vi "WPI_ADI_IMU_RefNum Registry Get.vi"(8 "error in (no error)":errorcluster, 11 "refnum name":string="ADIIMURefNum") -> (0 "error out":errorcluster, 3 "ADI IMU Interrupt DevRef":T1={"SimpleGyroDevRef"={"DevStatus"={"status"=FALSE, "code"=0, "source"=""}, "Handle"=0, "SPI Bus"=enum."SPI On-Board, CS0", "Device Found"=FALSE, "Sample Rate"=0.0, "Device Ready"=FALSE, "Yaw Axis"=enum."Z", "AHRS Algorithm"=enum."Complementary"}, "InterruptRef"={"DevStatus"={"status"=FALSE, "code"=0, "source"=""}, "InterruptIndex"=enum."0"}} {"SimpleGyroDevRef"."Sample Rate" min=0.25 max=100.0 step=0.25})   [LabVIEW 2015, in "FRC ADI MXP IMU.lvlib"]
doc: "Use this to get the reference you specify. You first must set the reference using RefNum Registry Set.vi."
uses:
  FRC ADI MXP IMU.lvlib
  WPI_AnalogDevicesIMUInterruptDevRef.ctl
  WPI_AnalogDevicesIMUDevRef.ctl
  <vilib>/Rock Robotics/SystemInterfaces/spilib/spi_bus.ctl
  <vilib>/Rock Robotics/WPI/Interrupt/WPI_InterruptRef.ctl
  <vilib>/Rock Robotics/SystemInterfaces/Interrupt/FPGA_InterruptIndex.ctl
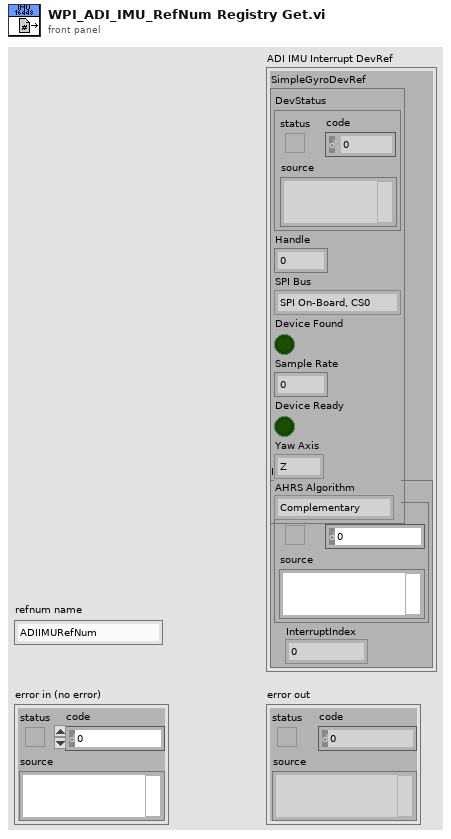
[diagram p1: front panel]
types:
  T1 = typedef "FRC ADI MXP IMU.lvlib/WPI_AnalogDevicesIMUInterruptDevRef.ctl" = cluster{"SimpleGyroDevRef":T2, "InterruptRef":T4}
  T2 = typedef "FRC ADI MXP IMU.lvlib/WPI_AnalogDevicesIMUDevRef.ctl" = cluster{"DevStatus":errorcluster, "Handle":i32, "SPI Bus":T3, "Device Found":bool, "Sample Rate":dbl, "Device Ready":bool, "Yaw Axis":enum16{"X", "Y", "Z"}, "AHRS Algorithm":enum16{"Complementary", "Madgwick"}}
  T3 = typedef "spi_bus.ctl" = enum16{"SPI On-Board, CS0", "SPI On-Board, CS1", "SPI On-Board, CS2", "SPI On-Board, CS3", "SPI MXP", "Invalid"}
  T4 = typedef "WPI_InterruptRef.ctl" = cluster{"DevStatus":errorcluster, "InterruptIndex":T5}
  T5 = typedef "FPGA_InterruptIndex.ctl" = enum8{"0", "1", "2", "3", "4", "5", "6", "7", "Invalid"}
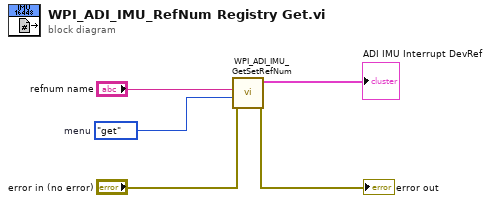
[diagram p0: block diagram]
diagram:
  w3 = enum16{"set", "get", "delete"}."get"  # menu
  n1 = call "WPI_ADI_IMU_GetSetRefNum.vi"("error in (no error)"="error in (no error)", "menu"=w3, "refnum name"="refnum name") -> ("error out"=→"error out":errorcluster, "ADI IMU Interrupt DevRef Get"=→"ADI IMU Interrupt DevRef":T1)  [unwired: 7 in]
